vi "Append Data.vi"(8 "error in (no error)":errorcluster, 9 "Check Data":bool[](array[boolean]), 10 "Cell Data":string[][](array[string]), 11 "MCListbox with Checkboxes in":refnum<class "MCListbox with Checkboxes.lvclass">) -> (0 "error out":errorcluster, 3 "MCListbox with Checkboxes out":refnum<class "MCListbox with Checkboxes.lvclass">)   [LabVIEW 2016, in "MCListbox with Checkboxes.lvclass"]
uses:
  MCListbox with Checkboxes.lvclass
  MCListbox with Checkboxes.lvclass/MCListbox with Checkboxes.ctl
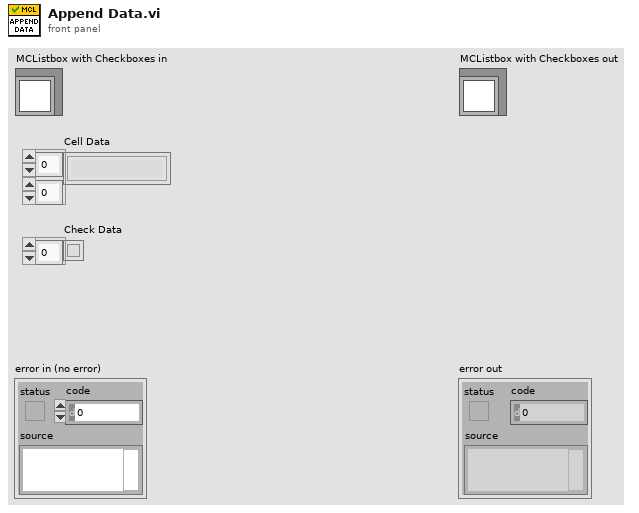
[diagram p1: front panel]
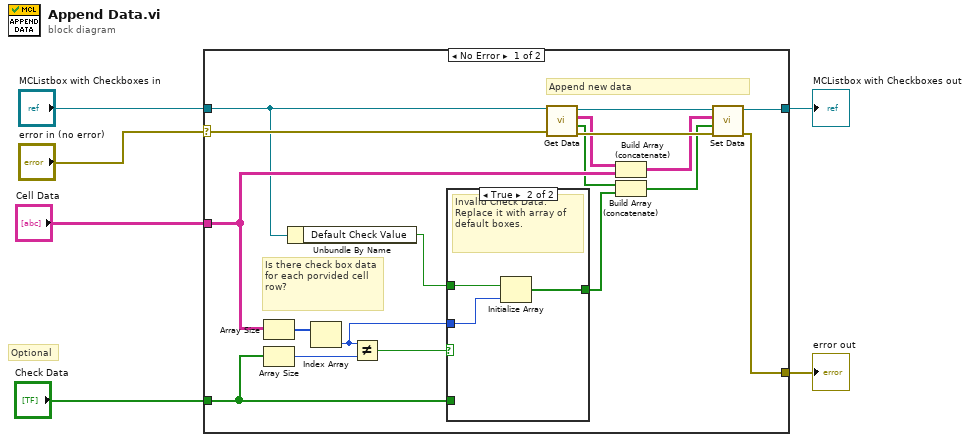
[diagram p0: block diagram]
diagram:
  # "Optional"
  n1 = case shown="No Error" "error in (no error)" {
    selector: "error in (no error)" -> [w23 w30]
    tunnel: [w12 w30] -> w5
    tunnel: [w13 w29] -> w3
    tunnel: "MCListbox with Checkboxes in" -> [w8 w29]
    tunnel: "Cell Data" -> [w19 _]
    tunnel: "Check Data" -> [w16 _]
    frame No Error {
      # "Is there check box data for each porvided cell row?"
      # "Append new data"
      n2 = Array Size(array=w19) -> (size(s)=w21:i32[])
      n3 = Array Size(array=w16) -> (size(s)=w20:i32)
      n4 = Unbundle By Name(w8) -> ("Default Check Value"=w7:bool)
      n5 = Index Array(array=w21) -> (element=w17:i32)  [unwired: 1 in]
      n6 = Not Equal?(x=w17, y=w20) -> (x != y?=w9:bool)
      n7 = case shown="True" w9 {
        tunnel: w17 -> [_ w28]
        tunnel: [w25 w27] -> w15
        tunnel: w16 -> [w25 _]
        tunnel: w7 -> [_ w26]
        frame False {
          # "Valid check data, use it."
        }
        frame True {
          # "Invalid Check Data. Replace it with array of default boxes."
          n8 = Initialize Array(w26, w28) -> (w27:bool[])
        }
      }
      n9 = call "Get Data.vi"("error in (no error)"=w23, "MCListbox with Checkboxes in"=w8) -> ("error out"=w24:errorcluster, "Check Data"=w18:bool[], "Cell Data"=w22:string[][], "MCListbox with Checkboxes out"=w14:refnum<class "MCListbox with Checkboxes.lvclass">)  [unwired: 6 in]
      n10 = Build Array (concatenate)(w22, w19) -> (w11:string[][])
      n11 = Build Array (concatenate)(w18, w15) -> (w10:bool[])
      n12 = call "Set Data.vi"("error in (no error)"=w24, "Check Data"=w10, "Cell Data"=w11, "MCListbox with Checkboxes in"=w14) -> ("error out"=w12:errorcluster, "MCListbox with Checkboxes out"=w13:refnum<class "MCListbox with Checkboxes.lvclass">)  [unwired: 6 in]
    }
    frame Error {
    }
  }
  "error out" <- w5
  "MCListbox with Checkboxes out" <- w3
